vi "ConvertToMode.vi"(1 "String":string) -> (0 "Numeric":i32)   [LabVIEW 2010]
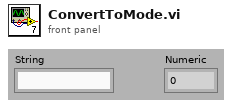
[diagram p1: front panel]
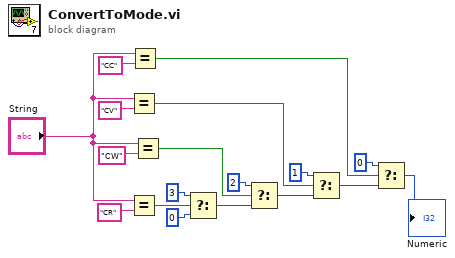
[diagram p0: block diagram]
diagram:
  n1 = Equal?(x="String", y="CV") -> (x = y?=w17:bool)
  n2 = Equal?(x="String", y="CR") -> (x = y?=w15:bool)
  n3 = Equal?(x="String", y="CC") -> (x = y?=w18:bool)
  n4 = Equal?(x="String", y="CW") -> (x = y?=w16:bool)
  n5 = Select(t=3, s=w15, f=0) -> (s? t:f=w6:i32)
  n6 = Select(t=2, s=w16, f=w6) -> (s? t:f=w7:i32)
  n7 = Select(t=1, s=w17, f=w7) -> (s? t:f=w8:i32)
  n8 = Select(t=0, s=w18, f=w8) -> (s? t:f=→"Numeric":i32)
